vi "run.create_set_property.vi"(8 "error in":errorcluster, 11 "RunCreateStaging in":refnum<class "RunCreateStaging.lvclass">) -> (0 "error out":errorcluster, 3 "RunCreateStaging out":refnum<class "RunCreateStaging.lvclass">)   [LabVIEW 2020, in "RunCreateStaging.lvclass"]
doc: "Sets a property (key/value pair) on the run being created."
uses:
  RunCreateStaging.lvclass
  RunCreateStaging.lvclass/RunCreateStaging.ctl
  client.lvlib
panel:
  in  "key":string
  in  "value":string
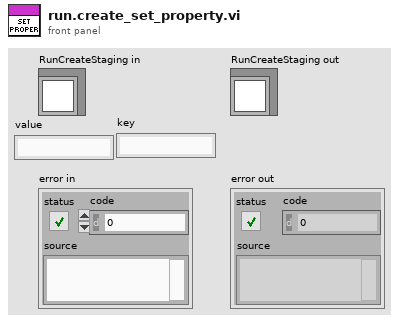
[diagram p1: front panel]
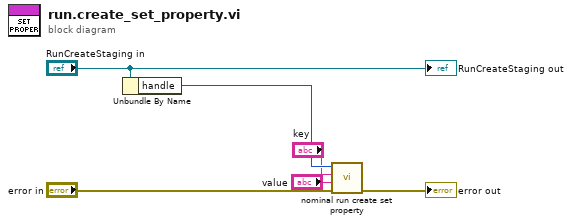
[diagram p0: block diagram]
diagram:
  n1 = Unbundle By Name("RunCreateStaging in") -> ("handle"=w4:i32)
  n2 = call "nominal run create set property.vi"("error in (no error)"="error in", "value"="value", "key"="key", "staging"=w4) -> ("error out"=→"error out":errorcluster)  [unwired: 6 in, 1 out]
  "RunCreateStaging out" <- "RunCreateStaging in"
